vi "Consumer.vi"(8 "error in (no error)":errorcluster, 9 "Data":variant, 10 "Case ID":string, 11 "uService Template in":refnum<class "Simple Device Manager.lvclass">) -> (0 "error out":errorcluster, 3 "uService Template out":refnum<class "Simple Device Manager.lvclass">)   [LabVIEW 2020, in "Simple Device Manager.lvlib" / "Simple Device Manager.lvclass"]
uses:
  Simple Device Manager.lvclass
  Consumer Case Selector.ctl
  Simple Device Manager.lvclass/Simple Device Manager.ctl
  Hardware/Simple Device/Simple Device.lvclass
  TALOS/TALOS_PPL.lvlibp/Father of all uServices/Father of all uServices/Father of all uServices.lvclass
  TALOS/TALOS_PPL.lvlibp
  C:/LabVIEW Code/aegis-labview-code/TALOS/TALOS_PPL.lvlibp/Father of all uServices/Father of all uServices/Father of all uServices.lvclass
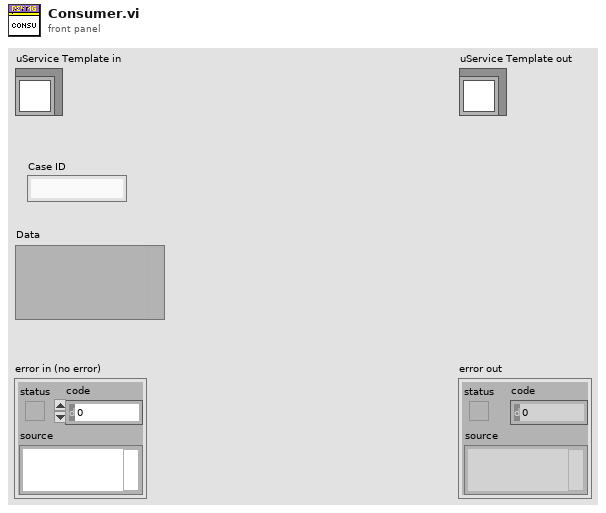
[diagram p1: front panel]
types:
  T1 = typedef "Simple Device Manager.lvlib/Simple Device Manager.lvclass/Consumer Case Selector.ctl" = enum16{"Set current", "Check status", "Check temperature"}
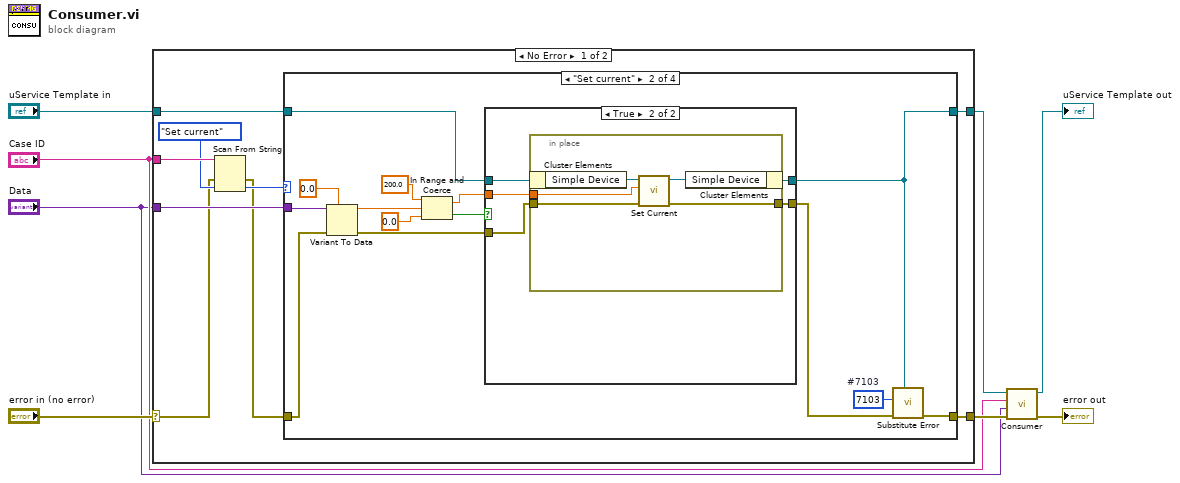
[diagram p0: block diagram]
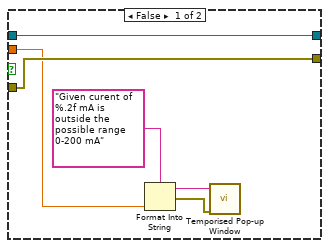
[diagram p3: hidden frame]
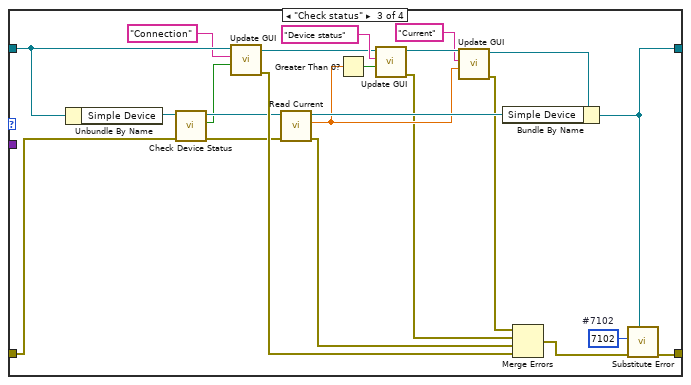
[diagram p4: hidden frame]
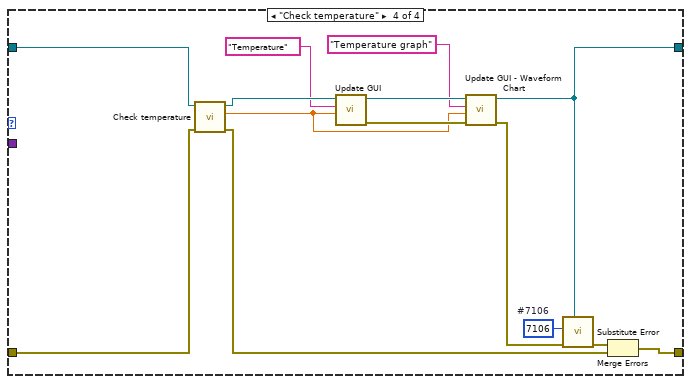
[diagram p5: hidden frame]
diagram:
  n1 = case shown="No Error" "error in (no error)" {
    selector: "error in (no error)" -> [w10 w87]
    tunnel: [w16 w88] -> w3
    tunnel: "uService Template in" -> [w17 w88]
    tunnel: [w14 w87] -> w6
    tunnel: "Case ID" -> [w13 _]
    tunnel: "Data" -> [w15 _]
    frame No Error {
      n2 = Scan From String(input string=w13, error in=w10, default 1=Consumer_Case_Selector."Set current" ("Consumer Case Selector")) -> (error out=w9:errorcluster, output 1=w11:T1)  [unwired: 2 in, 2 out]
      n3 = case shown="\"Set current\"" w11 {
        tunnel: w17 -> [w19 w30 w67 w86]
        tunnel: [w19 w21 w60 w77] -> w16
        tunnel: w15 -> [_ w33 _ _]
        tunnel: [w18 w22 w61 w80] -> w14
        tunnel: w9 -> [w18 w32 w71 w85]
        frame Default {
        }
        frame "Set current" {
          w20 = 7103  # #7103
          n4 = Variant To Data(error in=w32, type=0.0, Variant=w33) -> (data=w29:dbl, error out=w25:errorcluster)
          n5 = In Range and Coerce(upper limit=200.0, x=w29, lower limit=0.0) -> (coerced(x)=w24:dbl, In Range?=w26:bool)
          n6 = case shown="True" w26 {
            tunnel: [w38 w44] -> w23
            tunnel: [w39 w43] -> w21
            tunnel: w30 -> [w39 w42]
            tunnel: w25 -> [w38 w41]
            tunnel: w24 -> [w37 w40]
            frame False {
              n7 = Format Into String(format string="Given curent of %.2f mA is outside the possible range 0-200 mA", w37) -> (resulting string=w34:string, error out=w35:errorcluster)  [unwired: 2 in]
              n8 = call "Temporised Pop-up Window.vi"("error in (no error)"=w35, "Text"=w34) -> ()  [unwired: 9 in, 1 out]
            }
            frame True {
              n9 = in-place {
                in-place-border: w41 -> [w47]
                in-place-border: [w46] -> w44
                in-place-border: w40 -> [w45]
                n10 = in-place-cluster #1(w42) -> ("Simple Device"=w49:refnum<class "Simple Device.lvclass">)
                n11 = call-dynamic "Set Current.vi"("error in (no error)"=w47, "Current [mA]"=w45, "Simple Device in"=w49) -> ("error out"=w46:errorcluster, "Simple Device out"=w48:refnum<class "Simple Device.lvclass">)  [unwired: 7 in]
                n12 = in-place-cluster #1("Simple Device"=w48) -> (w43:refnum<class "Simple Device Manager.lvclass">)
              }
            }
          }
          n13 = call "Substitute Error.vi"("LabVIEW Object"=w21, "error in (no error)"=w23, "Error Code"=w20) -> ("error out"=w22:errorcluster)  [unwired: 8 in]
        }
        frame "Check status" {
          w55 = 7102  # #7102
          n14 = Unbundle By Name(w67) -> ("Simple Device"=w70:refnum<class "Simple Device.lvclass">)
          n15 = call-dynamic "Check Device Status.vi"("error in (no error)"=w71, "Simple Device in"=w70) -> ("error out"=w54:errorcluster, "Status"=w66:bool, "Simple Device out"=w69:refnum<class "Simple Device.lvclass">)  [unwired: 7 in]
          n16 = call "Update GUI.vi"("Data"=w66, "GUI Item Name"="Connection", "uService Template in"=w67) -> ("error out"=w72:errorcluster, "uService Template out"=w62:refnum<class "Simple Device Manager.lvclass">)  [unwired: 7 in]
          n17 = call-dynamic "Read Current.vi"("error in (no error)"=w54, "Simple Device in"=w69) -> ("error out"=w53:errorcluster, "Current [mA]"=w56:dbl, "Simple Device out"=w68:refnum<class "Simple Device.lvclass">)  [unwired: 7 in]
          n18 = Greater Than 0?(x=w56) -> (x > 0?=w64:bool)
          n19 = call "Update GUI.vi"("Data"=w64, "GUI Item Name"="Device status", "uService Template in"=w62) -> ("error out"=w52:errorcluster, "uService Template out"=w59:refnum<class "Simple Device Manager.lvclass">)  [unwired: 7 in]
          n20 = call "Update GUI.vi"("Data"=w56, "GUI Item Name"="Current", "uService Template in"=w59) -> ("error out"=w51:errorcluster, "uService Template out"=w58:refnum<class "Simple Device Manager.lvclass">)  [unwired: 7 in]
          n21 = Bundle By Name(cluster=w58, "Simple Device"=w68) -> (w60:refnum<class "Simple Device Manager.lvclass">)
          n22 = Merge Errors(w51, w52, w53, w72) -> (w50:errorcluster)
          n23 = call "Substitute Error.vi"("LabVIEW Object"=w60, "error in (no error)"=w50, "Error Code"=w55) -> ("error out"=w61:errorcluster)  [unwired: 8 in]
        }
        frame "Check temperature" {
          w73 = 7106  # #7106
          n24 = call-dynamic "Check temperature.vi"("error in (no error)"=w85, "Simple Device Manager in"=w86) -> ("error out"=w84:errorcluster, "Temperature"=w74:dbl, "Simple Device Manager out"=w81:refnum<class "Simple Device Manager.lvclass">)  [unwired: 7 in]
          n25 = call "Update GUI.vi"("Data"=w74, "GUI Item Name"="Temperature", "uService Template in"=w81) -> ("error out"=w82:errorcluster, "uService Template out"=w83:refnum<class "Simple Device Manager.lvclass">)  [unwired: 7 in]
          n26 = call "Update GUI - Waveform Chart.vi"("error in (no error)"=w82, "Point value"=w74, "GUI Item Name"="Temperature graph", "uService Template in"=w83) -> ("error out"=w78:errorcluster, "uService Template out"=w77:refnum<class "Simple Device Manager.lvclass">)  [unwired: 6 in]
          n27 = call "Substitute Error.vi"("LabVIEW Object"=w77, "error in (no error)"=w78, "Error Code"=w73) -> ("error out"=w79:errorcluster)  [unwired: 8 in]
          n28 = Merge Errors(w79, w84) -> (w80:errorcluster)
        }
      }
    }
    frame Error {
    }
  }
  n29 = call-parent "Consumer.vi"("error in (no error)"=w6, "Data"="Data", "Case ID"="Case ID", "uService Template in"=w3) -> ("error out"=→"error out":errorcluster, "uService Template out"=→"uService Template out":refnum<class "Simple Device Manager.lvclass">)  [unwired: 6 in]
